vi "filter.vi"(1 "peak indices":i32[](array[numeric]), 2 "FFT{x}":cdb[](array[numeric])) -> (0 "X":dbl[](array[numeric]))   [LabVIEW 2009]
uses:
  <vilib>/Analysis/2dsp.llb/Inverse Real FFT.vi
  <vilib>/Analysis/NI_AALPro.lvlib
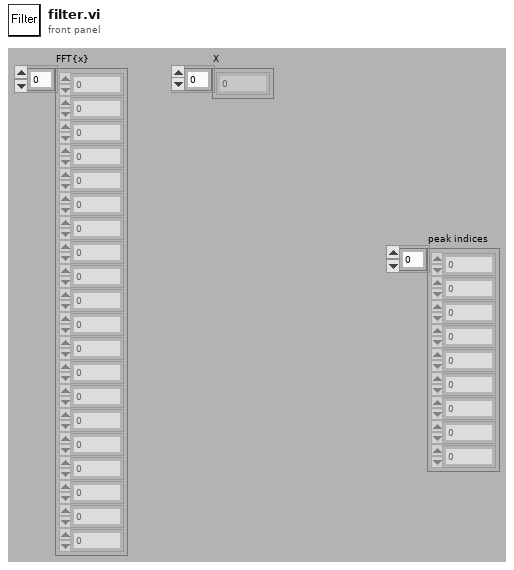
[diagram p1: front panel]
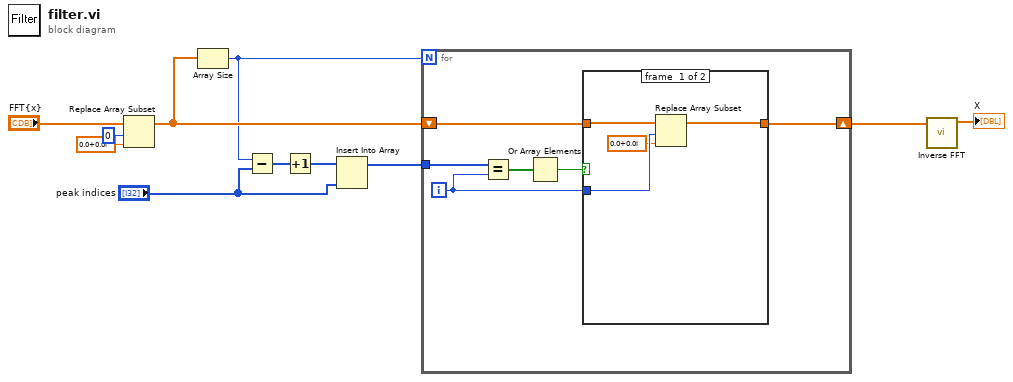
[diagram p0: block diagram]
diagram:
  n1 = Replace Array Subset(array="FFT{x}", new element=cdb 0.0+0.0i ("new element/subarray"), index=0) -> (w8:cdb[])
  n2 = Array Size(array=w8) -> (size(s)=w7:i32)
  n3 = Subtract(x=w7, y="peak indices") -> (x-y=w6:i32[])
  n4 = Increment(x=w6) -> (x+1=w5:i32[])
  n5 = Insert Into Array(array=w5, new element="peak indices") -> (w3:i32[])  [unwired: 1 in]
  n6 = for {
    N: w7 -> [_]
    shift-right: [w13] -> w2
    shift-left: w8 -> [w14]
    tunnel: w3 -> [w17]
    i -> [w12]
    n7 = Equal?(x=w17, y=w12) -> (x = y?=w16:bool[])
    n8 = Or Array Elements(Boolean array=w16) -> (logical OR=w15:bool)
    n9 = case shown="False" w15 {
      tunnel: w14 -> [w21 w22]
      tunnel: [w20 w22] -> w13
      tunnel: w12 -> [w19 _]
      frame #0 {
        n10 = Replace Array Subset(array=w21, new element=cdb 0.0+0.0i ("new element/subarray"), index=w19) -> (w20:cdb[])
      }
      frame #1 {
      }
    }
  }
  n11 = call-poly <vilib>:"Inverse FFT.vi"("FFT {X}"=w2) -> ("X"=→"X":dbl[])  [unwired: 9 in, 1 out]
